vi "filter_frequency_imp_test_v6.vi"() -> ()   [LabVIEW 2014]
uses:
  <vilib>/rvi/Analysis/host/Butterworth/config/Butterworth Filter Order.ctl
  <vilib>/rvi/Analysis/host/Butterworth/config/Butterworth Filter Type.ctl
  <vilib>/FPGAPlugInAG/cRIO-9039/niLvFpga_Open_cRIO-9039.vi
  <vilib>/rvi/interface/common/dynamic/niFpgaDynamicAddResources.vi
  <vilib>/rvi/Analysis/host/Butterworth/config/BwScaledCoefficients.vi
  <vilib>/Utility/error.llb/Error Cluster From Error Code.vi
  <vilib>/rvi/errors/niLvFpgaAdjustHostInterfaceError.vi
  <vilib>/FPGAPlugInAG/Dynamic/niLvFpga_Close_Dynamic.vi
  <vilib>/rvi/interface/nirviOpenFPGA/nirviOpenFPGA.xnode
  FPGA Bitfiles/test0304_FPGATarget_imptestv6_lu+KXd7CR6Y.lvbitx
  FPGA VIs/imp_test_v6.vi
  <vilib>/rvi/Analysis/host/Butterworth/XNode/ButterworthCoefficients.xnode
  <vilib>/rvi/interface/nirviReadWriteControl/nirviReadWriteControl.xnode
  <vilib>/rvi/interface/nirviCloseFPGA/nirviCloseFPGA.xnode
  <vilib>/rvi/Analysis/host/Public/NI_FpgaMspHost.lvlib
  NiFpgaLv.dll
  <vilib>/rvi/interface/Simulation/niFpgaSimulationCallBeginRW.vi
panel:
  in  "sr_Strain(Avg.8)_p (S/s)":dbl=50000.0
  in  "fcu_Strain(Avg.8)_p (Hz)":dbl=1000.0
  in  "sr_Strain(Avg.2)_y (S/s)":dbl=50000.0
  in  "fcu_Strain(Avg.2)_y (Hz)":dbl=1000.0
  in  "sr_Strain(Avg.4)_y (S/s)":dbl=50000.0
  in  "fcu_Strain(Avg.4)_y (Hz)":dbl=1000.0
  in  "sr_Dp_dd (S/s)":dbl=50000.0
  in  "fcu_Dp_dd (Hz)":dbl=1000.0
  in  "sr_dFp_PIS (S/s)":dbl=50000.0
  in  "fcu_dFp_PID (Hz)":dbl=1000.0
  in  "sr_Strain(Avg.8)_y (S/s)":dbl=50000.0
  in  "fcu_Strain(Avg.8)_y (Hz)":dbl=1000.0
  in  "sr_Dy_dd (S/s)":dbl=50000.0
  in  "fcu_Dy_dd (Hz)":dbl=1000.0
  in  "sr_dFy_PID (S/s)":dbl=50000.0
  in  "fcu_dFy_PID (Hz)":dbl=1000.0
  in  "stop":bool
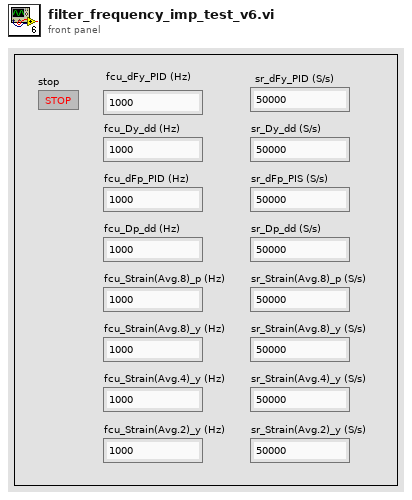
[diagram p1: front panel]
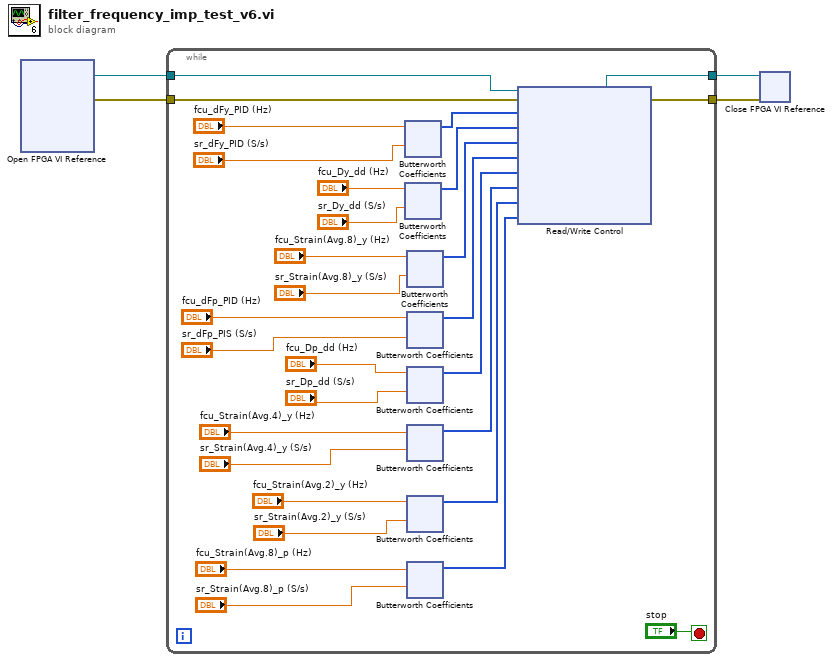
[diagram p0: block diagram]
diagram:
  n1 = xnode "Open FPGA VI Reference"() -> ("FPGA VI Reference Out"=w4:refnum<k20>, "error out"=w3:errorcluster)  [unwired: 2 in]
  n2 = while {
    tunnel: w4 -> [w24]
    tunnel: w3 -> [w33]
    tunnel: [w32] -> w2
    tunnel: [w31] -> w1
    stop <- "stop" stop-if-true
    n3 = xnode "Butterworth Coefficients"("cutoff frequency (Hz)"="fcu_dFy_PID (Hz)", "sample rate (S/s)"="sr_dFy_PID (S/s)") -> ("scaled coefficients"=w23:i32[])  [unwired: 1 in, 1 out]
    n4 = xnode "Butterworth Coefficients"("cutoff frequency (Hz)"="fcu_Dy_dd (Hz)", "sample rate (S/s)"="sr_Dy_dd (S/s)") -> ("scaled coefficients"=w22:i32[])  [unwired: 1 in, 1 out]
    n5 = xnode "Butterworth Coefficients"("cutoff frequency (Hz)"="fcu_Strain(Avg.8)_y (Hz)", "sample rate (S/s)"="sr_Strain(Avg.8)_y (S/s)") -> ("scaled coefficients"=w21:i32[])  [unwired: 1 in, 1 out]
    n6 = xnode "Butterworth Coefficients"("cutoff frequency (Hz)"="fcu_dFp_PID (Hz)", "sample rate (S/s)"="sr_dFp_PIS (S/s)") -> ("scaled coefficients"=w20:i32[])  [unwired: 1 in, 1 out]
    n7 = xnode "Butterworth Coefficients"("cutoff frequency (Hz)"="fcu_Dp_dd (Hz)", "sample rate (S/s)"="sr_Dp_dd (S/s)") -> ("scaled coefficients"=w19:i32[])  [unwired: 1 in, 1 out]
    n8 = xnode "Butterworth Coefficients"("cutoff frequency (Hz)"="fcu_Strain(Avg.4)_y (Hz)", "sample rate (S/s)"="sr_Strain(Avg.4)_y (S/s)") -> ("scaled coefficients"=w18:i32[])  [unwired: 1 in, 1 out]
    n9 = xnode "Butterworth Coefficients"("cutoff frequency (Hz)"="fcu_Strain(Avg.2)_y (Hz)", "sample rate (S/s)"="sr_Strain(Avg.2)_y (S/s)") -> ("scaled coefficients"=w10:i32[])  [unwired: 1 in, 1 out]
    n10 = xnode "Butterworth Coefficients"("cutoff frequency (Hz)"="fcu_Strain(Avg.8)_p (Hz)", "sample rate (S/s)"="sr_Strain(Avg.8)_p (S/s)") -> ("scaled coefficients"=w5:i32[])  [unwired: 1 in, 1 out]
    n11 = xnode "Read/Write Control"("FPGA VI Reference In"=w24, "error in"=w33, "dFy_PID coeff."=w23, "Dy_dd coeff."=w22, "Strain_y Avg8 coeff."=w21, "dFp_PID coeff."=w20, "Dp_dd coeff."=w19, "Strain_y Avg4 coeff."=w18, "Strain_y Avg2 coeff."=w10, "Strain_p Avg.8 coeff."=w5) -> ("FPGA VI Reference Out"=w32:refnum<k20>, "error out"=w31:errorcluster)
  }
  n12 = xnode "Close FPGA VI Reference"("FPGA VI Reference In"=w2, "error in"=w1) -> ()  [unwired: 1 out]
